vi "Dashboard Main.vi"() -> ()   [LabVIEW 2013]
uses:
  <vilib>/event_ctls.llb/eventvkey.ctl
  <vilib>/Rock Robotics/WPI/Dashboard/WPI_DashboardLogging Global.vi
  <vilib>/Utility/config.llb/Write Key (String).vi
  <vilib>/Utility/config.llb/Write Key (I32).vi
  <vilib>/Utility/config.llb/NI_LVConfig.lvlib
panel:
  in  "Camera Settings":T1={"Frame Rate"=30, "Compression"=30, "Size"=1} {"Frame Rate" scale=1.0..30.0; "Size" items=["640x480", "320x240", "160x120"]}
  out "fps":dbl format="%#.1g"
  out "Mbps":dbl format="%#.1g"
  out "Mbps 2":bool
  in  "DB Camera Config":bool
  out "Image Message":string="Timeout in Camera Communications"
  in  "Rec Mode":enum32{"Stop", "Record", "Playback"}(radio)
  in  "Dashboard Tab":T2(tab)
  out "Compressor Relay Status":bool
  out "Compressor Control Status":bool
  in  "Compressor Control":bool
  in  "Jag Position Enable":bool
  out "Right Direction Motor Position":dbl
  out "Left Direction Motor Position":dbl
  out "MotorSliders R":cluster{"MotorSlide1":dbl, "MotorSlide2":dbl} {"MotorSlide2" scale=-1.0..1.0 scale format="%#_2e"; "MotorSlide1" scale=-1.0..1.0 scale format="%#_2e"}
  out "MotorChart R":cluster{"Numeric":dbl, "Numeric":dbl}(graph)
  out "MotorSliders L":T3 {"MotorSlide4 2" scale=0.0..14.0 scale format="%#_2e"; "MotorSlide2" scale=-1.0..1.0 scale format="%#_2e"; "MotorSlide1" scale=-1.0..1.0 scale format="%#_2e"}
  out "MotorChart L":T4(graph)
  out "JS1 Z":dbl(slide) scale=-1.0..1.0 scale format="%#_2e"
  out "Joystick 1":cluster{"X":dbl, "Y":dbl}[](graph)
  out "JS Buttons 1":T5
  out "JS2 Z":dbl(slide) scale=-1.0..1.0 scale format="%#_2e"
  out "Joystick 2":cluster{"X":dbl, "Y":dbl}[](graph)
  out "JS Buttons 2":T5
  out "Mode":T6(ring)=enum."Auto Disabled"
  out "Camera IP":string
  in  "Test Slider":dbl(slide) scale=0.0..100.0 scale format="%#_3g"
  in  "On/Off":bool caption="Solenoid"
  in  "Test Name":u16(ring) items=["Select the test to run..."]
  in  "Test Tree":string(tree)
  in  "Motor":cluster{"Value":dbl, "Enable":bool} {"Value" scale=-1.0..1.0 scale format="%#_3g"}
  out "Progress":T7 {"Test Progress" scale=0.0..100.0}
  in  "Rev/Fwd":cluster{"Forward":bool, "Reverse":bool}
  in  "Test Ring":u16(ring) items=["Auto", "Fixed indoor", "Fixed outdoor 1", "Fixed outdoor 2", "Fixed fluorescent 1", "Fixed fluorescent 2", "Hold current"]
  in  "Listbox":i32(listbox)
  out "Tree":string(tree)
  out "Camera Image":T8(plugin-control)
  in  "Enable":bool
  # "Left"
  # "Right"
  # "Battery"
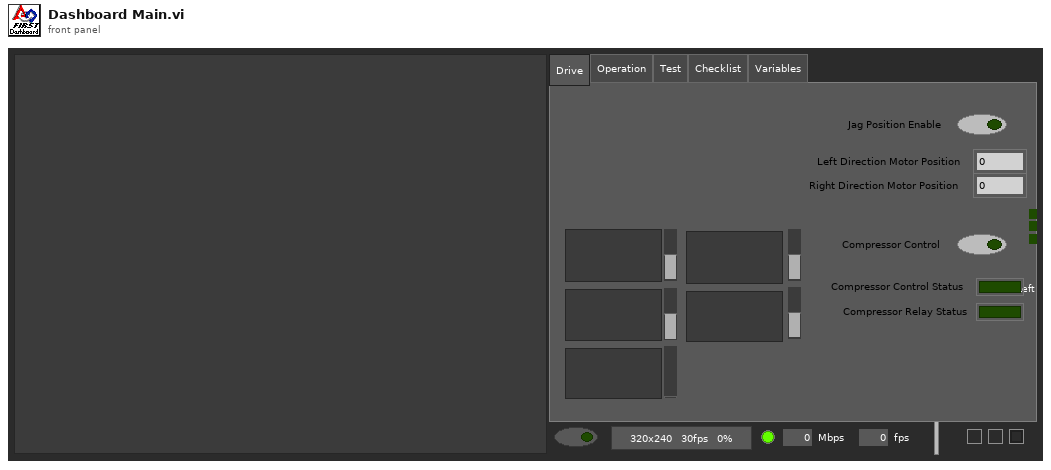
[diagram p1: front panel]
types:
  T1 = cluster{"Frame Rate":i32, "Compression":i32, "Size":u16}
  T2 = enum32{"Drive", "Operation", "Test", "Checklist", "Variables"}
  T3 = cluster{"MotorSlide1":dbl, "MotorSlide2":dbl, "MotorSlide4 2":dbl}
  T4 = cluster{"Numeric":dbl, "Numeric":dbl, "Battery":sgl}
  T5 = cluster{bool, bool, bool, bool, bool, bool, bool, bool, bool, bool, bool, bool}
  T6 = enum8{"Tele-Op Disabled", "Tele-Op Enabled", "Auto Disabled", "Auto Enabled", "Test Disabled", "Test Enabled", ""}
  T7 = cluster{"Test Progress":u8, "Test Progress Text":string}
  T8 = typedef "IMAQ Image.ctl" = refnum<image>
  T9 = enum32{"Drive", "Operation", "Auto", "Test", "Checklist", "Variables"}
  T10 = typedef "Image Type" = u32
  T11 = cluster{"Digital Inputs":bool[], "Digital Outputs":bool[]}
  T12 = cluster{"Competition mode":bool, "Robot Link":bool, "Autonomous":bool, "Enabled":bool, "E-Stop":bool, "Simulated":bool, "TestMode":bool, "Docked Window":bool}
  T13 = cluster{"Boolean Array[0]":bool, "Boolean Array[1]":bool, "Boolean Array[2]":bool, "Boolean Array[3]":bool, "Boolean Array[4]":bool, "Boolean Array[5]":bool, "Boolean Array[6]":bool, "Boolean Array[7]":bool, "Boolean Array[8]":bool, "Boolean Array[9]":bool, "Boolean Array[10]":bool, "Boolean Array[11]":bool}
  T14 = typedef "NI_LVConfig.lvlib/Config Data RefNum.ctl" = refnum<k1>
  T15 = typedef "eventvkey.ctl" = enum16{"ASCII", "Enter", "Return", "Shift", "Ctrl", "Alt", "Cmd", "Opt", "Caps", "NumLock", "Clear", "Break", "Up", "Down", "Left", "Right", "Insert", "Delete", "Home", "End", "PageUp", "PageDown", "Escape", "Help", "Pause", "ScrollLock", "F1", "F2", "F3", "F4", "F5", "F6", "F7", "F8", "F9", "F10", "F11", "F12", "F13", "F14", "F15", "F16", "F17", "F18", "F19", "F20", "F21", "F22", "F23", "F24", "Play", "VolumeUp", "VolumeDown", "Mute", "Two Byte Char"}
  T16 = cluster{"Image Size":bool, "Image Type":bool, "Pixel Value":bool, "ROI Information":bool, "Zoom Factor":bool}
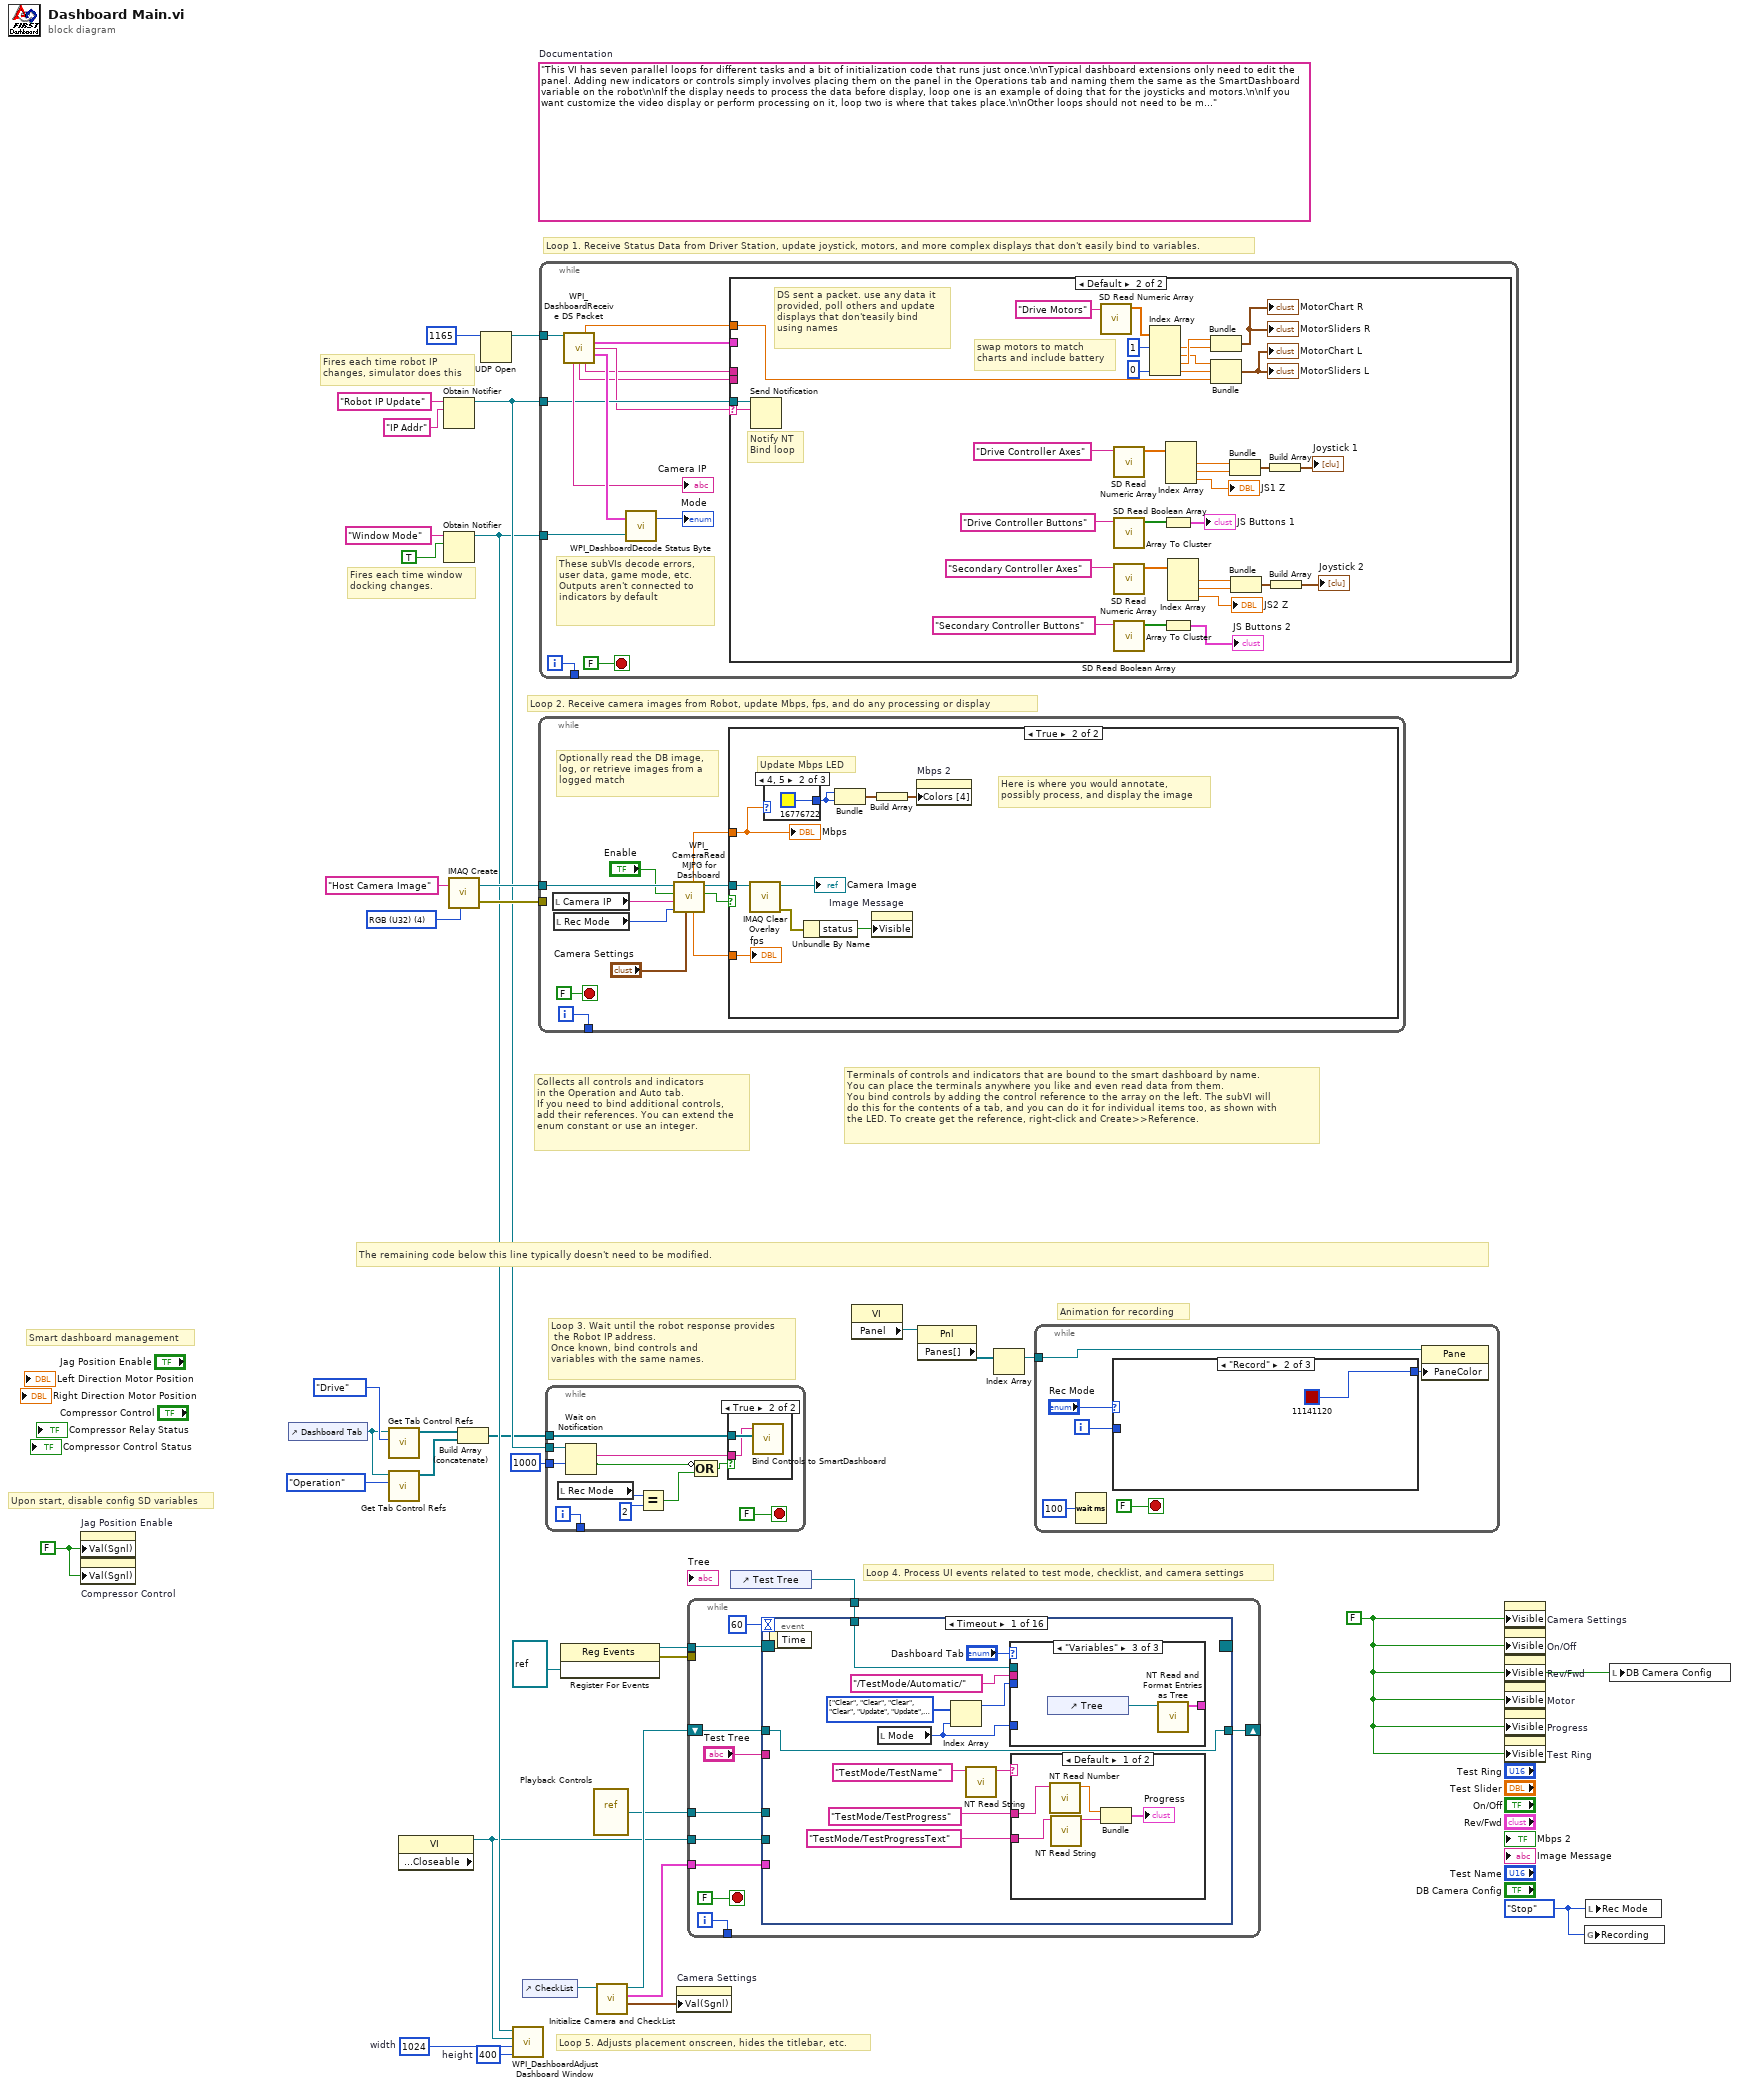
[diagram p0: block diagram]
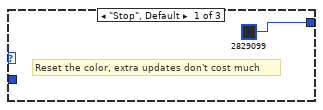
[diagram p2: hidden frame]
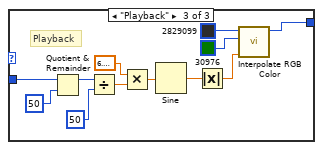
[diagram p3: hidden frame]
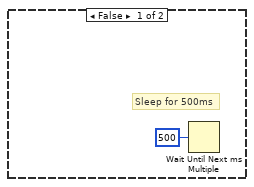
[diagram p5: hidden frame]
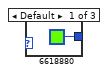
[diagram p6: hidden frame]
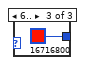
[diagram p7: hidden frame]
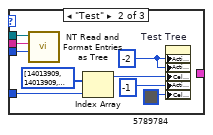
[diagram p9: hidden frame]
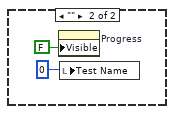
[diagram p10: hidden frame]
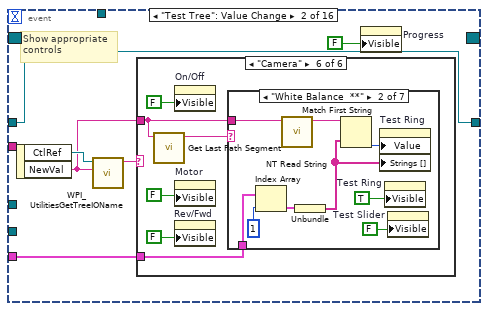
[diagram p11: hidden frame]
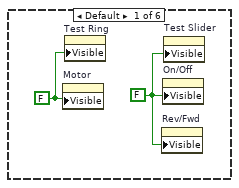
[diagram p12: hidden frame]
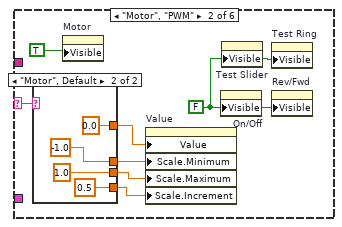
[diagram p13: hidden frame]
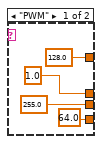
[diagram p14: hidden frame]
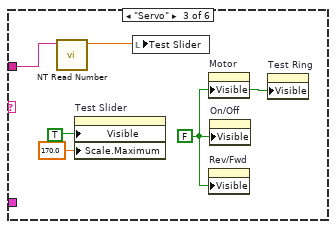
[diagram p15: hidden frame]
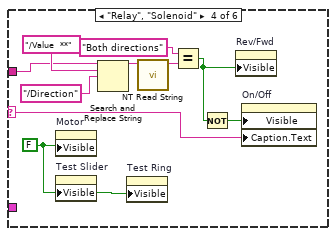
[diagram p16: hidden frame]
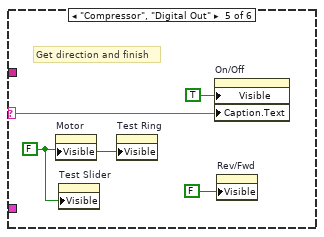
[diagram p17: hidden frame]
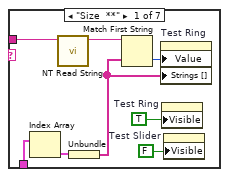
[diagram p18: hidden frame]
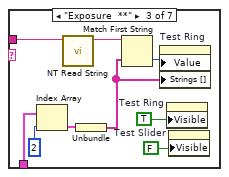
[diagram p19: hidden frame]
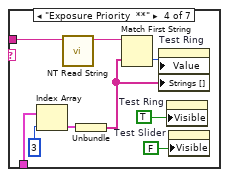
[diagram p20: hidden frame]
diagram:
  w1 = FALSE ("Value (Signaling)")
  w8 = enum32{"Stop", "Record", "Playback"}."Stop" ("Rec Mode")
  w11 = 400  # height
  w12 = 1024  # width
  w25 = FALSE ("Visible")
  (unwired) "This VI has seven parallel loops for different tasks and a bit of initialization code that runs just once.\n\nTypical dashboard extensions only need to edit the panel. Adding new indicators or controls simply involves placing them on the panel in the Operations tab and naming them the same as the SmartDashboard variable on the robot\n\nIf the display needs to process the data before display, loop one is an example of doing that for the joysticks and motors.\n\nIf you want customize the video display or perform processing on it, loop two is where that takes place.\n\nOther loops should not need to be modified. They are pretty standard, and document the task they perform."  # Documentation
  w35 = T10 4 items=["Grayscale (U8)", "Grayscale (I16)", "Grayscale (SGL)", "Complex (CSG)", "RGB (U32)", "HSL (U32)", "RGB (U64)"] ("Image Type")
  # "Upon start, disable config SD variables"
  # "Smart dashboard management"
  # "Animation for recording"
  # "Fires each time robot IP\nchanges, simulator does this"
  # "Fires each time window\ndocking changes."
  # "Collects all controls and indicators\nin the Operation and Auto tab.\nIf you need to bind additional controls,\nadd their references. You can extend the\nenum constant or use an integer."
  # "The remaining code below this line typically doesn't need to be modified."
  # "Loop 4. Process UI events related to test mode, checklist, and camera settings"
  # "Terminals of controls and indicators that are bound to the smart dashboard by name.\nYou can place the terminals anywhere you like and even read data from them.\nYou bind controls by adding the control reference to the array on the left. The subVI will\ndo this for the contents of a tab, and you can do it for individual items too, as shown with\nthe LED. To create get the reference, right-click and Create>>Reference."
  # "Loop 3. Wait until the robot response provides\n the Robot IP address.\nOnce known, bind controls and\nvariables with the same names."
  # "Loop 5. Adjusts placement onscreen, hides the titlebar, etc."
  # "Loop 1. Receive Status Data from Driver Station, update joystick, motors, and more complex displays that don't easily bind to variables."
  # "Loop 2. Receive camera images from Robot, update Mbps, fps, and do any processing or display"
  n1 = property on="Jag Position Enable" class="Bool (strict)"("Val(Sgnl)"=w1) -> ()  [unwired: 2 in, 2 out]
  n2 = property on="Compressor Control" class="Bool (strict)"("Val(Sgnl)"=w1) -> ()  [unwired: 2 in, 2 out]
  n3 = control-ref of="Dashboard Tab"() -> (w6:refnum<vi>)
  n4 = call <vilib>:"Get Tab Control Refs.vi"("Page Index"=T9."Drive" ("Dashboard Tab"), "TabControl in"=w6) -> ("ControlsOnPage"=w4:refnum<vi>[])  [unwired: 9 in]
  n5 = call <vilib>:"Get Tab Control Refs.vi"("Page Index"=T9."Operation" ("Dashboard Tab"), "TabControl in"=w6) -> ("ControlsOnPage"=w5:refnum<vi>[])  [unwired: 9 in]
  n6 = property class="VI" props=["Front Panel.Closeable"]() -> (reference out=w7:refnum<vi>)  [unwired: 2 in, 2 out]
  n7 = Obtain Notifier(name (unnamed)="Robot IP Update", notification data type="IP Addr" ("name (unnamed)")) -> (notifier out=w29:refnum<notifier>)  [unwired: 2 in, 2 out]
  n8 = Obtain Notifier(name (unnamed)="Window Mode", notification data type=TRUE) -> (notifier out=w10:refnum<notifier>)  [unwired: 2 in, 2 out]
  n9 = call "IMAQ Create"("Image Name"="Host Camera Image", "Image Type"=w35) -> ("New Image"=w33:T8, "error out"=w32:errorcluster)  [unwired: 2 in, 1 out]
  n10 = Build Array (concatenate)(w4, w5) -> (w3:refnum<vi>[])
  n11 = UDP Open(11:u16 1165 ("port")) -> (port=w36:refnum<k16>)  [unwired: 2 in, 4 out]
  n12 = call <vilib>:"WPI_DashboardAdjust Dashboard Window.vi"("height"=w11, "width"=w12, "reference in"=w7, "Notifier in"=w10) -> ()  [unwired: 8 in]
  n13 = control-ref of="CheckList"() -> (w9:refnum<vi>)
  n14 = while {
    tunnel: w33 -> [w46]
    tunnel: w32 -> [_]
    tunnel: [w47] -> _
    i -> [w47]
    stop <- FALSE stop-if-true
    # "Optionally read the DB image,\nlog, or retrieve images from a\nlogged match"
    n15 = local read "Camera IP"() -> (w39:string)
    n16 = local read "Rec Mode"() -> (w38:enum32{"Stop", "Record", "Playback"})
    n17 = call <vilib>:"WPI_CameraRead MJPG for Dashboard.vi"("Camera Settings"="Camera Settings", "Rec Mode"=w38, "Camera IP"=w39, "Enable"="Enable", "Refnum in"=w46) -> ("Active"=w43:bool, "Refnum out"=w45:T8, "FPS"=w42:dbl, "Bandwidth (Mbps)"=w41:dbl)  [unwired: 3 in]
    n18 = case shown="True" w43 {
      tunnel: w45 -> [_ w53]
      tunnel: w41 -> [_ w52]
      tunnel: w42 -> [_ w50]
      frame False {
        # "Sleep for 500ms"
        n19 = Wait Until Next ms Multiple(millisecond multiple=u32 500) -> ()  [unwired: 1 out]
      }
      frame True {
        # "Here is where you would annotate,\npossibly process, and display the image"
        # "Update Mbps LED"
        n20 = call "IMAQ Clear Overlay"("Image"=w53) -> ("error out"=w57:errorcluster, "Image Out"=→"Camera Image":T8)  [unwired: 2 in, 7 out]
        n21 = case shown="4, 5" w52 {
          tunnel: [u32 6618880 ("Color Box") u32 16776722 ("Color Box") u32 16716800 ("Color Box")] -> w54
          frame Default {
          }
          frame 4, 5 {
          }
          frame 6.. {
          }
        }
        n22 = Unbundle By Name(w57) -> ("status"=w58:bool)
        n23 = Bundle("Color Box"=w54, "Color Box"=w54) -> (w56:cluster{"Color Box":u32, "Color Box":u32})  [unwired: 1 out]
        n24 = property on="Image Message" class="Str"("Visible"=w58) -> ()  [unwired: 2 in, 2 out]
        n25 = Build Array(w56) -> (w55:cluster{"Color Box":u32, "Color Box":u32}[])
        n26 = property on="Mbps 2" class="Bool (strict)"("Colors [4]"=w55) -> ()  [unwired: 2 in, 2 out]
        "Mbps" <- w52
        "fps" <- w50
      }
    }
  }
  n27 = while {
    tunnel: w36 -> [w72]
    tunnel: w29 -> [w67]
    tunnel: w10 -> [w71]
    tunnel: [w68] -> _
    i -> [w68]
    stop <- FALSE stop-if-true
    # "These subVIs decode errors, user data, game mode, etc.\nOutputs aren't connected to indicators by default"
    n28 = call <vilib>:"WPI_DashboardReceive DS Packet.vi"("Recv Socket"=w72) -> ("Battery"=w62:sgl, "Driver Station"=w63:T11, "Robot IP Address"=w66:string, "Status"=w73:T12, "Camera IP Address"=→"Camera IP":string, "Low Priority User Data"=w65:string, "High Priority User Data"=w64:string)  [unwired: 1 in, 7 out]
    n29 = call <vilib>:"WPI_DashboardDecode Status Byte.vi"("Window Mode Notifier"=w71, "Status"=w73) -> ("Mode"=→"Mode":T6)  [unwired: 1 out]
    n30 = case shown="Default" w66 {
      selector: w66 -> [_ w85]
      tunnel: w67 -> [_ w86]
      tunnel: w65 -> [_ _]
      tunnel: w64 -> [_ _]
      tunnel: w63 -> [_ _]
      tunnel: w62 -> [_ w84]
      frame "0.0.0.0" {
        # "DS not sending packets, or no robot exists yet.\nDon't poll the variables"
      }
      frame Default {
        # "Notify NT\nBind loop"
        # "DS sent a packet. use any data it\nprovided, poll others and update\ndisplays that don'teasily bind\nusing names"
        # "swap motors to match\ncharts and include battery"
        n31 = Send Notification(notification=w85, notifier=w86) -> ()  [unwired: 1 in, 2 out]
        n32 = call <vilib>:"SD Read Numeric Array.vi"("Name"="Drive Motors") -> ("Numeric Array"=w83:dbl[])  [unwired: 8 in, 2 out]
        n33 = call <vilib>:"SD Read Numeric Array.vi"("Name"="Drive Controller Axes") -> ("Numeric Array"=w102:dbl[])  [unwired: 8 in, 2 out]
        n34 = call <vilib>:"SD Read Boolean Array.vi"("Name"="Drive Controller Buttons") -> ("Boolean Array"=w104:bool[])  [unwired: 8 in, 2 out]
        n35 = call <vilib>:"SD Read Numeric Array.vi"("Name"="Secondary Controller Axes") -> ("Numeric Array"=w96:dbl[])  [unwired: 8 in, 2 out]
        n36 = call <vilib>:"SD Read Boolean Array.vi"("Name"="Secondary Controller Buttons") -> ("Boolean Array"=w95:bool[])  [unwired: 8 in, 2 out]
        n37 = Index Array(array=w83, index #1=1, index #4=0) -> (element #1=w79:dbl, element #2=w78:dbl, element #3=w80:dbl, element #4=w75:dbl)  [unwired: 2 in]
        n38 = Array To Cluster(array=w104) -> (cluster=→"JS Buttons 1":T13)
        n39 = Array To Cluster(array=w95) -> (cluster=→"JS Buttons 2":T13)
        n40 = Index Array(array=w102) -> (element #1=w99:dbl, element #2=w100:dbl, element #3=→"JS1 Z":dbl)  [unwired: 3 in]
        n41 = Index Array(array=w96) -> (element #1=w91:dbl, element #2=w90:dbl, element #3=→"JS2 Z":dbl)  [unwired: 3 in]
        n42 = Bundle("Numeric"=w80, "Numeric"=w79) -> (→"MotorChart R" →"MotorSliders R":cluster{"Numeric":dbl, "Numeric":dbl})  [unwired: 1 in]
        n43 = Bundle("Numeric"=w78, "Numeric"=w75, "Battery"=w84) -> (→"MotorChart L" →"MotorSliders L":T4)  [unwired: 1 in]
        n44 = Bundle("Numeric"=w99, "Numeric"=w100) -> (w98:cluster{"Numeric":dbl, "Numeric":dbl})  [unwired: 1 in]
        n45 = Bundle("Numeric"=w91, "Numeric"=w90) -> (w92:cluster{"Numeric":dbl, "Numeric":dbl})  [unwired: 1 in]
        n46 = Build Array(w98) -> (→"Joystick 1":cluster{"Numeric":dbl, "Numeric":dbl}[])
        n47 = Build Array(w92) -> (→"Joystick 2":cluster{"Numeric":dbl, "Numeric":dbl}[])
      }
    }
  }
  n48 = while {
    tunnel: w3 -> [w118]
    tunnel: w29 -> [w116]
    tunnel: [w114] -> _
    tunnel: u32 1000 ("milliseconds to wait") -> [w113]
    i -> [w114]
    stop <- FALSE stop-if-true
    n49 = local read "Rec Mode"() -> (w109:enum32{"Stop", "Record", "Playback"})
    n50 = Wait on Notification(notifier=w116, timeout in ms (-1)=w113) -> (notification=w115:string, timed out?=w111:bool)  [unwired: 2 in, 2 out]
    n51 = Equal?(x=w109, y=u16 2 ("Rec Mode")) -> (x = y?=w110:bool)
    n52 = Compound Arithmetic op=OR(invert w111, w110) -> (w112:bool)
    n53 = case shown="True" w112 {
      tunnel: w118 -> [_ w120]
      tunnel: w115 -> [_ w119]
      frame False {
      }
      frame True {
        n54 = call <vilib>:"Bind Controls to SmartDashboard.vi"("Bound Control Refs"=w120, "Server IP Address"=w119) -> ()  [unwired: 10 in]
      }
    }
  }
  n55 = register-events(refnum<vi> refnum) -> (reference out=w16:refnum<event-registration>, error out=w15:errorcluster)  [unwired: 2 in]
  n56 = vi-ref "Playback Controls.vi"() -> (w17:refnum<vi>)
  n57 = call "Initialize Camera and CheckList.vi"("ListBox in"=w9) -> ("Cluster"=w23:cluster{"value":i32, "value":i32, "index":i32}, "Array"=w24:cluster{string[]}[], "File Refnum"=w22:T14)  [unwired: 8 in]
  n58 = property on="Camera Settings" class="Clust (strict)"("Val(Sgnl)"=w23) -> ()  [unwired: 2 in, 2 out]
  n59 = control-ref of="Test Tree"() -> (w21:refnum<vi>)
  n60 = while {
    tunnel: w24 -> [w128]
    shift-right: [w127] -> _
    shift-left: w22 -> [w126]
    tunnel: [w125] -> _
    tunnel: w21 -> [w124]
    tunnel: w17 -> [w123]
    tunnel: w16 -> [w122]
    tunnel: w15 -> [_]
    tunnel: w7 -> [w121]
    i -> [w125]
    stop <- FALSE stop-if-true
    n61 = event shown="[0] Timeout" {
      selector: w122 -> [_ _ _ _ _ _ _ _ _ _ _ _ _ _ _ _]
      dyn-events: [_ _ _ _ _ _ _ _ _ _ _ _ _ w366 _ _] -> _
      timeout: u32 60 ("milliseconds to wait") -> [_ _ _ _ _ _ _ _ _ _ _ _ _ _ _ _]
      tunnel: w124 -> [w138 _ _ _ _ _ _ _ _ _ _ _ _ _ _ _]
      tunnel: "Test Tree" -> [_ _ _ _ _ _ _ _ w335 w343 w345 w349 w357 _ _ _]
      tunnel: w128 -> [_ w162 _ _ _ _ w299 w329 _ _ _ _ _ _ _ _]
      tunnel: [w132 w161 w260 w265 w273 w285 w298 w322 w334 w341 w344 w348 w356 w368 w382 w383] -> w127
      tunnel: w126 -> [w132 w161 w260 w265 w273 w285 w297 w322 w334 w341 w344 w348 w356 w368 w382 w383]
      tunnel: w123 -> [_ _ _ _ _ _ _ _ _ _ _ _ _ w369 _ w386]
      tunnel: w121 -> [_ _ _ _ _ _ _ _ _ _ _ _ _ w364 _ _]
      event Timeout {
        w137 = enum16{"Update", "Clear"}[] [enum."Clear", enum."Clear", enum."Clear", enum."Clear", enum."Update", enum."Update", enum."Clear"] items=["Update", "Clear"]
        n62 = event-data() -> ()  [unwired: 1 in, 1 out]
        n63 = local read "Mode"() -> (w135:T6)
        n64 = Index Array(array=w137, index=w135) -> (element=w136:enum16{"Update", "Clear"})
        n65 = call <vilib>:"NT Read String.vi"("Name"="TestMode/TestName") -> ("String"=w141:string)  [unwired: 9 in, 1 out]
        n66 = case shown="\"Variables\"" "Dashboard Tab" {
          tunnel: w138 -> [_ w151 _]
          tunnel: "/TestMode/Automatic/" ("Name Pattern") -> [_ w150 _]
          tunnel: w136 -> [_ w149 _]
          tunnel: w135 -> [_ w147 _]
          tunnel: [_ _ w153] -> _
          frame "Operation", Default {
          }
          frame "Test" {
            w146 = -2 ("Active Item:Row Number")
            n67 = call <vilib>:"NT Read and Format Entries as Tree.vi"("Operation"=w149, "Name Pattern"=w150, "Tree Refnum"=w151) -> ()  [unwired: 7 in, 2 out]
            n68 = Index Array(array=u32[] [14013909, 14013909, 14013909, 14013909, 14013909, 16777215, 14013909], index=w147) -> (element=w145:u32)
            n69 = property on="Test Tree" class="Tree (strict)"("Active Item Row Number"=w146, "ActiveColNum"=w146, "CellBG"=w145, "Active Item Row Number"=-1 ("Active Item:Row Number"), "CellBG"=u32 5789784 ("Color Box")) -> ()  [unwired: 2 in, 2 out]
          }
          frame "Variables" {
            n70 = control-ref of="Tree"() -> (w152:refnum<vi>)
            n71 = call <vilib>:"NT Read and Format Entries as Tree.vi"("Tree Refnum"=w152) -> ("Formatted Strings"=w153:cluster{"Name":string, "Value":string}[])  [unwired: 9 in, 1 out]
          }
        }
        n72 = case shown="Default" w141 {
          tunnel: "TestMode/TestProgress" ("Name") -> [w155 _]
          tunnel: "TestMode/TestProgressText" ("Name") -> [w154 _]
          frame Default {
            n73 = call <vilib>:"NT Read Number.vi"("Name"=w155) -> ("Numeric"=w156:dbl)  [unwired: 9 in, 1 out]
            n74 = call <vilib>:"NT Read String.vi"("Name"=w154) -> ("String"=w157:string)  [unwired: 9 in, 1 out]
            n75 = Bundle("Numeric"=w156, "String"=w157) -> (→"Progress":cluster{"Numeric":dbl, "String":string})  [unwired: 1 in]
          }
          frame "" {
            n76 = property on="Progress" class="Clust (strict)"("Visible"=FALSE) -> ()  [unwired: 2 in, 2 out]
            n77 = local write "Test Name"(u16 0) -> ()
          }
        }
      }
      event "Test Tree": Value Change {
        # "Show appropriate\ncontrols"
        n78 = event-data() -> ("CtlRef"=w165:refnum<vi>, "NewVal"=w163:string)  [unwired: 1 in]
        n79 = call <vilib>:"WPI_UtilitiesGetTreeIOName.vi"("NewVal"=w163, "TreeControl in"=w165) -> ("I/O Name"=w166:string)  [unwired: 9 in]
        n80 = case shown="\"Camera\"" w166 {
          selector: w166 -> [_ w173 _ w191 w200 _]
          tunnel: w163 -> [_ _ w188 w190 _ w207]
          tunnel: w162 -> [_ _ _ _ _ w206]
          frame Default {
            w168 = FALSE ("Visible")
            w167 = FALSE ("Visible")
            n81 = property on="Motor" class="Clust (strict)"("Visible"=w167) -> ()  [unwired: 2 in, 2 out]
            n82 = property on="Test Ring" class="Ring (strict)"("Visible"=w167) -> ()  [unwired: 2 in, 2 out]
            n83 = property on="Rev/Fwd" class="Clust (strict)"("Visible"=w168) -> ()  [unwired: 2 in, 2 out]
            n84 = property on="On/Off" class="Bool (strict)"("Visible"=w168) -> ()  [unwired: 2 in, 2 out]
            n85 = property on="Test Slider" class="Slide (strict)"("Visible"=w168) -> ()  [unwired: 2 in, 2 out]
          }
          frame "Motor", "PWM" {
            w174 = FALSE ("Visible")
            n86 = case shown="\"Motor\", Default" w173 {
              tunnel: [1.0 ("Value") -1.0 ("Value")] -> w172
              tunnel: [255.0 ("Value") 1.0 ("Value")] -> w171
              tunnel: [128.0 ("Value") 0.0 ("Value")] -> w170
              tunnel: [64.0 ("Value") 0.5 ("Value")] -> w169
              frame "PWM" {
              }
              frame "Motor", Default {
              }
            }
            n87 = property on="Motor" class="Clust (strict)"("Visible"=TRUE) -> ()  [unwired: 2 in, 2 out]
            n88 = property on="Value" class="Slide (strict)"("Value"=w170, "Scale.Minimum"=w172, "Scale.Maximum"=w171, "Scale.Increment"=w169) -> ()  [unwired: 2 in, 2 out]
            n89 = property on="On/Off" class="Bool (strict)"("Visible"=w174) -> ()  [unwired: 2 in, 2 out]
            n90 = property on="Test Slider" class="Slide (strict)"("Visible"=w174) -> ()  [unwired: 2 in, 2 out]
            n91 = property on="Test Ring" class="Ring (strict)"("Visible"=w174) -> ()  [unwired: 2 in, 2 out]
            n92 = property on="Rev/Fwd" class="Clust (strict)"("Visible"=w174) -> ()  [unwired: 2 in, 2 out]
          }
          frame "Servo" {
            w186 = FALSE ("Visible")
            n93 = call <vilib>:"NT Read Number.vi"("Name"=w188) -> ("Numeric"=w187:dbl)  [unwired: 9 in, 1 out]
            n94 = property on="Test Slider" class="Slide (strict)"("Visible"=TRUE, "Scale.Maximum"=170.0 ("Scale.Range:Maximum")) -> ()  [unwired: 2 in, 2 out]
            n95 = local write "Test Slider"(w187) -> ()
            n96 = property on="Motor" class="Clust (strict)"("Visible"=w186) -> ()  [unwired: 2 in, 2 out]
            n97 = property on="Rev/Fwd" class="Clust (strict)"("Visible"=w186) -> ()  [unwired: 2 in, 2 out]
            n98 = property on="On/Off" class="Bool (strict)"("Visible"=w186) -> ()  [unwired: 2 in, 2 out]
            n99 = property on="Test Ring" class="Ring (strict)"("Visible"=w186) -> ()  [unwired: 2 in, 2 out]
          }
          frame "Relay", "Solenoid" {
            w189 = FALSE ("Visible")
            n100 = property on="Motor" class="Clust (strict)"("Visible"=w189) -> ()  [unwired: 2 in, 2 out]
            n101 = property on="Test Slider" class="Slide (strict)"("Visible"=w189) -> ()  [unwired: 2 in, 2 out]
            n102 = Search and Replace String(input string=w190, search string="/Value  **", replace string="/Direction") -> (result string=w196:string)  [unwired: 5 in, 3 out]
            n103 = property on="Test Ring" class="Ring (strict)"("Visible"=w189) -> ()  [unwired: 2 in, 2 out]
            n104 = call <vilib>:"NT Read String.vi"("Name"=w196) -> ("String"=w194:string)  [unwired: 9 in, 1 out]
            n105 = Equal?(x="Both directions", y=w194) -> (x = y?=w192:bool)
            n106 = Not(x=w192) -> (.not. x?=w193:bool)
            n107 = property on="Rev/Fwd" class="Clust (strict)"("Visible"=w192) -> ()  [unwired: 2 in, 2 out]
            n108 = property on="On/Off" class="Bool (strict)"("Visible"=w193, "Caption.Text"=w191) -> ()  [unwired: 2 in, 2 out]
          }
          frame "Compressor", "Digital Out" {
            w199 = FALSE ("Visible")
            # "Get direction and finish"
            n109 = property on="Motor" class="Clust (strict)"("Visible"=w199) -> ()  [unwired: 2 in, 2 out]
            n110 = property on="Test Slider" class="Slide (strict)"("Visible"=w199) -> ()  [unwired: 2 in, 2 out]
            n111 = property on="Test Ring" class="Ring (strict)"("Visible"=w199) -> ()  [unwired: 2 in, 2 out]
            n112 = property on="On/Off" class="Bool (strict)"("Visible"=TRUE, "Caption.Text"=w200) -> ()  [unwired: 2 in, 2 out]
            n113 = property on="Rev/Fwd" class="Clust (strict)"("Visible"=FALSE) -> ()  [unwired: 2 in, 2 out]
          }
          frame "Camera" {
            n114 = call <vilib>:"Get Last Path Segment.vi"("String in"=w207) -> ("String out"=w208:string)  [unwired: 10 in]
            n115 = property on="On/Off" class="Bool (strict)"("Visible"=FALSE) -> ()  [unwired: 2 in, 2 out]
            n116 = property on="Motor" class="Clust (strict)"("Visible"=FALSE) -> ()  [unwired: 2 in, 2 out]
            n117 = property on="Rev/Fwd" class="Clust (strict)"("Visible"=FALSE) -> ()  [unwired: 2 in, 2 out]
            n118 = case shown="\"White Balance  **\"" w208 {
              tunnel: w207 -> [w214 w223 w232 w241 w250 _ w256]
              tunnel: w206 -> [w212 w220 w229 w238 w247 _ _]
              frame "Size  **" {
                n119 = Index Array(array=w212) -> (element=w211:cluster{string[]})  [unwired: 1 in]
                n120 = call <vilib>:"NT Read String.vi"("Name"=w214) -> ("String"=w213:string)  [unwired: 9 in, 1 out]
                n121 = Unbundle(w211) -> (w209:string[])
                n122 = Match First String(2:w209, 3:w213) -> (0:w210:i32)  [unwired: 1 out]
                n123 = property on="Test Ring" class="Ring (strict)"("Value"=w210, "Strings []"=w209) -> ()  [unwired: 2 in, 2 out]
                n124 = property on="Test Ring" class="Ring (strict)"("Visible"=TRUE) -> ()  [unwired: 2 in, 2 out]
                n125 = property on="Test Slider" class="Slide (strict)"("Visible"=FALSE) -> ()  [unwired: 2 in, 2 out]
              }
              frame "White Balance  **" {
                n126 = Index Array(array=w220, index=1) -> (element=w221:cluster{string[]})
                n127 = call <vilib>:"NT Read String.vi"("Name"=w223) -> ("String"=w222:string)  [unwired: 9 in, 1 out]
                n128 = Unbundle(w221) -> (w218:string[])
                n129 = Match First String(2:w218, 3:w222) -> (0:w217:i32)  [unwired: 1 out]
                n130 = property on="Test Ring" class="Ring (strict)"("Value"=w217, "Strings []"=w218) -> ()  [unwired: 2 in, 2 out]
                n131 = property on="Test Ring" class="Ring (strict)"("Visible"=TRUE) -> ()  [unwired: 2 in, 2 out]
                n132 = property on="Test Slider" class="Slide (strict)"("Visible"=FALSE) -> ()  [unwired: 2 in, 2 out]
              }
              frame "Exposure  **" {
                n133 = Index Array(array=w229, index=2) -> (element=w230:cluster{string[]})
                n134 = call <vilib>:"NT Read String.vi"("Name"=w232) -> ("String"=w231:string)  [unwired: 9 in, 1 out]
                n135 = Unbundle(w230) -> (w226:string[])
                n136 = Match First String(2:w226, 3:w231) -> (0:w227:i32)  [unwired: 1 out]
                n137 = property on="Test Ring" class="Ring (strict)"("Value"=w227, "Strings []"=w226) -> ()  [unwired: 2 in, 2 out]
                n138 = property on="Test Ring" class="Ring (strict)"("Visible"=TRUE) -> ()  [unwired: 2 in, 2 out]
                n139 = property on="Test Slider" class="Slide (strict)"("Visible"=FALSE) -> ()  [unwired: 2 in, 2 out]
              }
              frame "Exposure Priority  **" {
                n140 = Index Array(array=w238, index=3) -> (element=w239:cluster{string[]})
                n141 = call <vilib>:"NT Read String.vi"("Name"=w241) -> ("String"=w240:string)  [unwired: 9 in, 1 out]
                n142 = Unbundle(w239) -> (w235:string[])
                n143 = Match First String(2:w235, 3:w240) -> (0:w236:i32)  [unwired: 1 out]
                n144 = property on="Test Ring" class="Ring (strict)"("Value"=w236, "Strings []"=w235) -> ()  [unwired: 2 in, 2 out]
                n145 = property on="Test Ring" class="Ring (strict)"("Visible"=TRUE) -> ()  [unwired: 2 in, 2 out]
                n146 = property on="Test Slider" class="Slide (strict)"("Visible"=FALSE) -> ()  [unwired: 2 in, 2 out]
              }
              frame "Color Enable  **" {
                n147 = Index Array(array=w247, index=4) -> (element=w248:cluster{string[]})
                n148 = call <vilib>:"NT Read String.vi"("Name"=w250) -> ("String"=w249:string)  [unwired: 9 in, 1 out]
                n149 = Unbundle(w248) -> (w244:string[])
                n150 = Match First String(2:w244, 3:w249) -> (0:w245:i32)  [unwired: 1 out]
                n151 = property on="Test Ring" class="Ring (strict)"("Value"=w245, "Strings []"=w244) -> ()  [unwired: 2 in, 2 out]
                n152 = property on="Test Ring" class="Ring (strict)"("Visible"=TRUE) -> ()  [unwired: 2 in, 2 out]
                n153 = property on="Test Slider" class="Slide (strict)"("Visible"=FALSE) -> ()  [unwired: 2 in, 2 out]
              }
              frame Default {
                n154 = property on="Test Ring" class="Ring (strict)"("Visible"=FALSE) -> ()  [unwired: 2 in, 2 out]
                n155 = property on="Test Slider" class="Slide (strict)"("Visible"=FALSE) -> ()  [unwired: 2 in, 2 out]
              }
              frame "Brightness  **", "Color Level  **", "Compression  **", "FPS  **", "Sharpness  **" {
                n156 = call <vilib>:"NT Read Number.vi"("Name"=w256) -> ("Numeric"=w255:dbl)  [unwired: 9 in, 1 out]
                n157 = local write "Test Slider"(w255) -> ()
                n158 = property on="Test Slider" class="Slide (strict)"("Visible"=TRUE, "Scale.Maximum"=100.0 ("Scale.Range:Maximum")) -> ()  [unwired: 2 in, 2 out]
                n159 = property on="Test Ring" class="Ring (strict)"("Visible"=FALSE) -> ()  [unwired: 2 in, 2 out]
              }
            }
          }
        }
        n160 = property on="Progress" class="Clust (strict)"("Visible"=FALSE) -> ()  [unwired: 2 in, 2 out]
      }
      event "Test Name": Mouse Enter {
        # "Populate the ring with the list of tests"
        n161 = event-data() -> ()  [unwired: 1 in, 1 out]
        n162 = call <vilib>:"NT Read String Array.vi"("Name"="TestMode/TestList") -> ("String Array"=w264:string[])  [unwired: 9 in, 1 out]
        n163 = Build Array (concatenate)("Select the test to run...", w264) -> (w263:string[])
        n164 = property on="Test Name" class="Ring (strict)"("Strings []"=w263) -> ()  [unwired: 2 in, 2 out]
      }
      event "Test Name": Value Change {
        w266 = FALSE ("Visible")
        # "Tell the robot the test name to run"
        n165 = event-data() -> ("NewVal"=w270:u16)  [unwired: 1 in]
        n166 = property on="Test Name" class="Ring (strict)"() -> ("Strings []"=w271:string[])  [unwired: 2 in, 2 out]
        n167 = local write "Progress"(T7 {"Test Progress"=0, "Test Progress Text"=""} ("Progress")) -> ()
        n168 = Index Array(array=w271, index=w270) -> (element=w269:string)
        n169 = call <vilib>:"NT Write String.vi"("String"=w269, "Name"="TestMode/TestName") -> ()  [unwired: 9 in, 1 out]
        n170 = property on="Progress" class="Clust (strict)"("Visible"=TRUE) -> ()  [unwired: 2 in, 2 out]
        n171 = property on="Motor" class="Clust (strict)"("Visible"=w266) -> ()  [unwired: 2 in, 2 out]
        n172 = property on="Test Slider" class="Slide (strict)"("Visible"=w266) -> ()  [unwired: 2 in, 2 out]
        n173 = property on="On/Off" class="Bool (strict)"("Visible"=w266) -> ()  [unwired: 2 in, 2 out]
        n174 = property on="Rev/Fwd" class="Clust (strict)"("Visible"=w266) -> ()  [unwired: 2 in, 2 out]
        n175 = property on="Test Ring" class="Ring (strict)"("Visible"=w266) -> ()  [unwired: 2 in, 2 out]
      }
      event "Listbox": Double Click {
        n176 = event-data() -> ("PlatMods.Shift"=w274:bool, "Row"=w276:i32)  [unwired: 1 in]
        n177 = case shown="True" w274 {
          tunnel: w276 -> [w280 _]
          tunnel: 1 -> [w279 _]
          frame False {
            n178 = property on="Listbox" class="LstBox (strict)"() -> ("Item Symbols"=w278:i32[])  [unwired: 2 in, 2 out]
            n179 = Replace Array Subset(array=w278, new element=w279, index=w280) -> (w277:i32[])
            n180 = property on="Listbox" class="LstBox (strict)"("Item Symbols"=w277) -> ()  [unwired: 2 in, 2 out]
          }
          frame True {
            w281 = 0 ("Top Row")
            n181 = property on="Listbox" class="LstBox (strict)"() -> ("Number of Rows"=w283:u32)  [unwired: 2 in, 2 out]
            n182 = Initialize Array(0, w283) -> (w282:i32[])
            n183 = property on="Listbox" class="LstBox (strict)"("Top Row"=w281, "Value"=w281, "Item Symbols"=w282) -> ()  [unwired: 2 in, 2 out]
          }
        }
      }
      event "Listbox": Key Down {
        n184 = event-data() -> ("VKey"=w287:T15)  [unwired: 1 in]
        n185 = case shown="\"Left\", \"Right\"" w287 {
          selector: w287 -> [w292 _]
          tunnel: eventvkey."Left" ("VKey") -> [w290 _]
          frame "Left", "Right" {
            n186 = Equal?(x=w290, y=w292) -> (x = y?=w291:bool)
            n187 = Select(t=0, s=w291, f=1) -> (s? t:f=w293:i32)
            n188 = property on="Listbox" class="LstBox (strict)"() -> ("Item Symbols"=w296:i32[])  [unwired: 2 in, 2 out]
            n189 = Replace Array Subset(array=w296, new element=w293, index="Listbox") -> (w295:i32[])
            n190 = property on="Listbox" class="LstBox (strict)"("Item Symbols"=w295) -> ()  [unwired: 2 in, 2 out]
          }
          frame Default {
          }
        }
      }
      event "DB Camera Config": Value Change {
        n191 = event-data() -> ("NewVal"=w300:bool)  [unwired: 1 in]
        n192 = case shown="False" w300 {
          tunnel: w299 -> [w309 _]
          tunnel: [w302 w320] -> w298
          tunnel: w297 -> [w301 w320]
          frame False {
            w316 = "Camera"
            w319 = FALSE ("Visible")
            n193 = local read "Camera Settings"() -> (w308:T1)
            n194 = Index Array(array=w309) -> (element=w312:cluster{string[]})  [unwired: 1 in]
            n195 = Unbundle(w308) -> ("Frame Rate"=w307:i32, "Compression"=w306:i32, "Size"=w310:u16)
            n196 = Unbundle(w312) -> (w311:string[])
            n197 = Index Array(array=w311, index=w310) -> (element=w305:string)
            n198 = call-poly <vilib>:"Write Key.vi"("section"=w316, "value"=w305, "key"="Size", "refnum"=w301) -> ("refnum out"=w318:T14)  [unwired: 2 in, 5 out]
            n199 = call-poly <vilib>:"Write Key.vi"("section"=w316, "value"=w307, "key"="FrameRate", "refnum"=w318) -> ("refnum out"=w317:T14)  [unwired: 1 in, 6 out]
            n200 = property on="Camera Settings" class="Clust (strict)"("Visible"=w319) -> ()  [unwired: 2 in, 2 out]
            n201 = local write "DB Camera Config"(w319) -> ()
            n202 = call-poly <vilib>:"Write Key.vi"("section"=w316, "value"=w306, "key"="Compression", "refnum"=w317) -> ("refnum out"=w303:T14)  [unwired: 1 in, 6 out]
            n203 = call <vilib>:"Close Config Data.vi"("refnum"=w303) -> ("file path"=w304:path)  [unwired: 2 in, 8 out]
            n204 = call <vilib>:"Open Config Data.vi"("configuration file path"=w304) -> ("refnum"=w302:T14)  [unwired: 8 in, 2 out]
          }
          frame True {
            n205 = property on="Camera Settings" class="Clust (strict)"("Visible"=TRUE) -> ()  [unwired: 2 in, 2 out]
          }
        }
      }
      event "Camera Settings": Value Change {
        n206 = event-data() -> ("NewVal"=w333:T1)  [unwired: 1 in]
        n207 = Index Array(array=w329) -> (element=w328:cluster{string[]})  [unwired: 1 in]
        n208 = Unbundle(w333) -> ("Frame Rate"=w324:i32, "Compression"=w323:i32, "Size"=w326:u16)
        n209 = Unbundle(w328) -> (w327:string[])
        n210 = Index Array(array=w327, index=w326) -> (element=w325:string)
        n211 = Format Into String(format string="%s   %dfps   %d%%", w325, w324, w323) -> (resulting string=w330:string)  [unwired: 2 in, 1 out]
        n212 = Build Array(w330) -> (w331:string[])
        n213 = property on="DB Camera Config" class="Bool (strict)"("Strings [4]"=w331) -> ()  [unwired: 2 in, 2 out]
      }
      event "Motor.Enable": Value Change {
        n214 = event-data() -> ("NewVal"=w339:bool)  [unwired: 1 in]
        n215 = Unbundle("Motor") -> ("Value"=w338:dbl)  [unwired: 1 out]
        n216 = Select(t=w338, s=w339, f=0.0) -> (s? t:f=w336:dbl)
        n217 = call <vilib>:"NT Write Number.vi"("Numeric"=w336, "Name"=w335) -> ()  [unwired: 9 in, 1 out]
      }
      event "Test Slider": Value Change {
        n218 = event-data() -> ("NewVal"=w342:dbl)  [unwired: 1 in]
        n219 = call <vilib>:"NT Write Number.vi"("Numeric"=w342, "Name"=w343) -> ()  [unwired: 9 in, 1 out]
      }
      event "On/Off": Value Change {
        n220 = event-data() -> ("NewVal"=w347:bool)  [unwired: 1 in]
        n221 = Boolean To (0,1)(Boolean=w347) -> (0, 1=w346:i16)
        n222 = call <vilib>:"NT Write Number.vi"("Numeric"=w346, "Name"=w345) -> ()  [unwired: 9 in, 1 out]
      }
      event "Rev/Fwd": Value Change {
        n223 = event-data() -> ("NewVal.Forward"=w355:bool, "NewVal.Reverse"=w354:bool)  [unwired: 1 in]
        n224 = Boolean To (0,1)(Boolean=w355) -> (0, 1=w351:i16)
        n225 = Boolean To (0,1)(Boolean=w354) -> (0, 1=w353:i16)
        n226 = Negate(x=w353) -> (-x=w352:i16)
        n227 = Add(x=w351, y=w352) -> (x+y=w350:i16)
        n228 = call <vilib>:"NT Write Number.vi"("Numeric"=w350, "Name"=w349) -> ()  [unwired: 9 in, 1 out]
      }
      event "Test Ring": Value Change {
        n229 = event-data() -> ("NewVal"=w359:u16)  [unwired: 1 in]
        n230 = property on="Test Ring" class="Ring (strict)"() -> ("Strings []"=w360:string[])  [unwired: 2 in, 2 out]
        n231 = Index Array(array=w360, index=w359) -> (element=w358:string)
        n232 = call <vilib>:"NT Write String.vi"("String"=w358, "Name"=w357) -> ()  [unwired: 9 in, 1 out]
      }
      event "Rec Mode": Value Change {
        # "Update globals for recording mode and path to read log from.\nClear when logging and let NetworkTables set path for vision to\nuse."
        n233 = event-data() -> ("NewVal"=w370:enum32{"Stop", "Record", "Playback"})  [unwired: 1 in]
        n234 = global write "WPI_DashboardLogging Global.vi" "Logging Filename"(path "") -> ()
        n235 = case shown="\"Stop\", \"Record\"" w370 {
          tunnel: w369 -> [_ w372 w380]
          tunnel: [_ _ w379] -> w366
          tunnel: [_ _ w378] -> _
          tunnel: w364 -> [_ _ w376]
          tunnel: cluster{i32, i32} {-250, 170} -> [_ _ w375]
          tunnel: [_ _ T16 {"Image Size"=TRUE, "Image Type"=TRUE, "Pixel Value"=TRUE, "ROI Information"=TRUE, "Zoom Factor"=FALSE} ("Image Information Shown:All Elements")] -> w362
          tunnel: [_ _ TRUE ("Zoom Factor")] -> w361
          frame Default {
          }
          frame "Stop", "Record" {
            # "Place Window too"
            n236 = invoke class="VI" method="FP.Close"(reference=w372) -> (reference out=w371:refnum<vi>)  [unwired: 2 in, 2 out]
            n237 = invoke class="VI" method="Abort VI"(reference=w371) -> ()  [unwired: 2 in, 3 out]
          }
          frame "Playback" {
            n238 = call "Open Playback Panel.vi"("Offset"=w375, "DB VI Ref"=w376, "Playback in"=w380) -> ("Playback out"=w377:refnum<vi>)  [unwired: 8 in]
            n239 = register-events(w377) -> (reference out=w379:refnum<event-registration>, error out=w378:errorcluster)  [unwired: 2 in]
          }
        }
        n240 = global write "WPI_DashboardLogging Global.vi" "Recording"(w370) -> ()
        n241 = property on="Camera Image" class="ImageControl"("Image Information Shown"=w362, "Image Information Visible"=w361) -> ()  [unwired: 2 in, 2 out]
        n242 = call <vilib>:"WPI_DashboardNT Log FieldName Cache.vi"("Operation"=enum16{"Lookup/Add", "Index", "Clear"}."Clear") -> ()  [unwired: 8 in, 3 out]
      }
      event Panel Close {
        w381 = enum32{"Stop", "Record", "Playback"}."Stop" ("Rec Mode")
        n243 = event-data() -> ()  [unwired: 1 in, 4 out]
        n244 = local write "Rec Mode"(w381) -> ()
        n245 = global write "WPI_DashboardLogging Global.vi" "Recording"(w381) -> ()
      }
      event Panel Close {
        # "Abort playback window and ourself"
        n246 = event-data() -> ()  [unwired: 1 in, 4 out]
        n247 = invoke class="VI" method="FP.Close"(reference=w386) -> (reference out=w385:refnum<vi>)  [unwired: 2 in, 2 out]
        n248 = invoke class="VI" method="Abort VI"(reference=w385) -> (error out=w384:errorcluster)  [unwired: 2 in, 2 out]
        n249 = invoke class="VI" method="Abort VI"(error in=w384) -> ()  [unwired: 2 in, 3 out]
      }
    }
  }
  n250 = property class="VI"() -> ("Panel"=w19:refnum<vi>)  [unwired: 2 in, 2 out]
  n251 = property class="Pnl"(reference=w19) -> ("Panes[]"=w20:refnum<vi>[])  [unwired: 1 in, 2 out]
  n252 = Index Array(array=w20) -> (element=w18:refnum<vi>)  [unwired: 1 in]
  n253 = while {
    tunnel: w18 -> [w388]
    i -> [w391]
    stop <- FALSE stop-if-true
    n254 = Wait (ms)(milliseconds to wait=u32 100) -> ()  [unwired: 1 out]
    n255 = case shown="\"Record\"" "Rec Mode" {
      tunnel: w391 -> [_ _ w406]
      tunnel: [u32 2829099 ("Base Color") u32 11141120 ("Target Color") w395] -> w387
      frame "Stop", Default {
        # "Reset the color, extra updates don't cost much"
      }
      frame "Record" {
      }
      frame "Playback" {
        # "Playback"
        n256 = Quotient & Remainder(x=w406, y=u32 50 ("milliseconds to wait")) -> (x-y*floor(x/y)=w402:u32)  [unwired: 1 out]
        n257 = Divide(x=w402, y=u32 50 ("milliseconds to wait")) -> (x/y=w399:dbl)
        n258 = Multiply(x=6.283185307179586, y=w399) -> (x*y=w404:dbl)
        n259 = Sine(x=w404) -> (sin(x)=w403:dbl)
        n260 = Absolute Value(x=w403) -> (abs(x)=w396:dbl)
        n261 = call "Interpolate RGB Color.vi"("Proportion"=w396, "Target Color"=u32 30976, "Base Color"=u32 2829099) -> ("Result Color"=w395:u32)  [unwired: 8 in]
      }
    }
    n262 = property class="Pane"(reference=w388, "PaneColor"=w387) -> ()  [unwired: 1 in, 2 out]
  }
  n263 = property on="Camera Settings" class="Clust (strict)"("Visible"=w25) -> ()  [unwired: 2 in, 2 out]
  n264 = property on="On/Off" class="Bool (strict)"("Visible"=w25) -> ()  [unwired: 2 in, 2 out]
  n265 = property on="Rev/Fwd" class="Clust (strict)"("Visible"=w25) -> ()  [unwired: 2 in, 2 out]
  n266 = property on="Motor" class="Clust (strict)"("Visible"=w25) -> ()  [unwired: 2 in, 2 out]
  n267 = property on="Progress" class="Clust (strict)"("Visible"=w25) -> ()  [unwired: 2 in, 2 out]
  n268 = property on="Test Ring" class="Ring (strict)"("Visible"=w25) -> ()  [unwired: 2 in, 2 out]
  n269 = global write "WPI_DashboardLogging Global.vi" "Recording"(w8) -> ()
  n270 = local write "Rec Mode"(w8) -> ()
  n271 = local write "DB Camera Config"(w25) -> ()
